vi "I2C Grove AlphaNumeric LED.vi"() -> ()   [LabVIEW 2020, in "CTI-Scratchpad.lvlib"]
uses:
  CTI-Scratchpad.lvlib
  CTI/Identity.ctl
  CTI/Error Reporting.ctl
  CTI/I2C Address.ctl
  CTI/GPIO Number.ctl
  CTI/I2C Number.ctl
  CTI/Session/Session.lvclass
  CTI-Peripheral/LEDAlphaNumeric/HT16K33 LED Driver/HT16K33 LED Driver.lvclass
  CTI/VisaComms/VisaComms.lvclass
  CTI/CTI.lvlib
panel:
  in  "Numeric In":string
  in  "Set Numeric":bool
  in  "String":string
  in  "Set Char":bool
  out "Identity":T1
  in  "stop":bool
  in  "Grove Connector":enum16{"I2C0", "I2C1"}(ring)
  out "error out":errorcluster
  in  "Port":refnum<visa-resource-name>="COM4"
  # "https://wiki.seeedstudio.com/Grove-0.54_inch_Red_Quad_Alphanumeric_Display/"
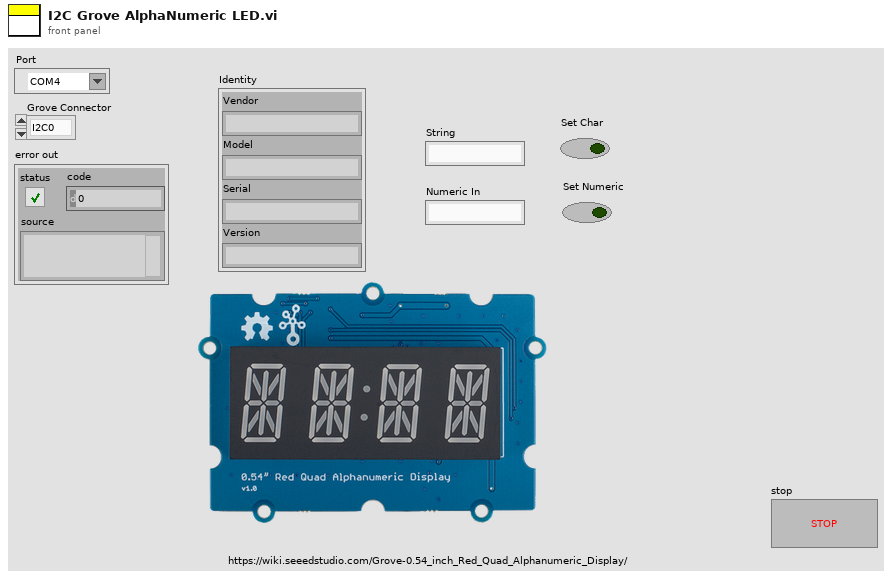
[diagram p1: front panel]
types:
  T1 = typedef "CTI.lvlib/Identity.ctl" = cluster{"Vendor":string, "Model":string, "Serial":string, "Version":string}
  T2 = typedef "CTI.lvlib/I2C Address.ctl" = u8
  T3 = typedef "CTI.lvlib/Error Reporting.ctl" = enum16{"Minimal", "Moderate", "Full"}
  T4 = typedef "CTI.lvlib/I2C Number.ctl" = i8
  T5 = typedef "CTI.lvlib/GPIO Number.ctl" = i8
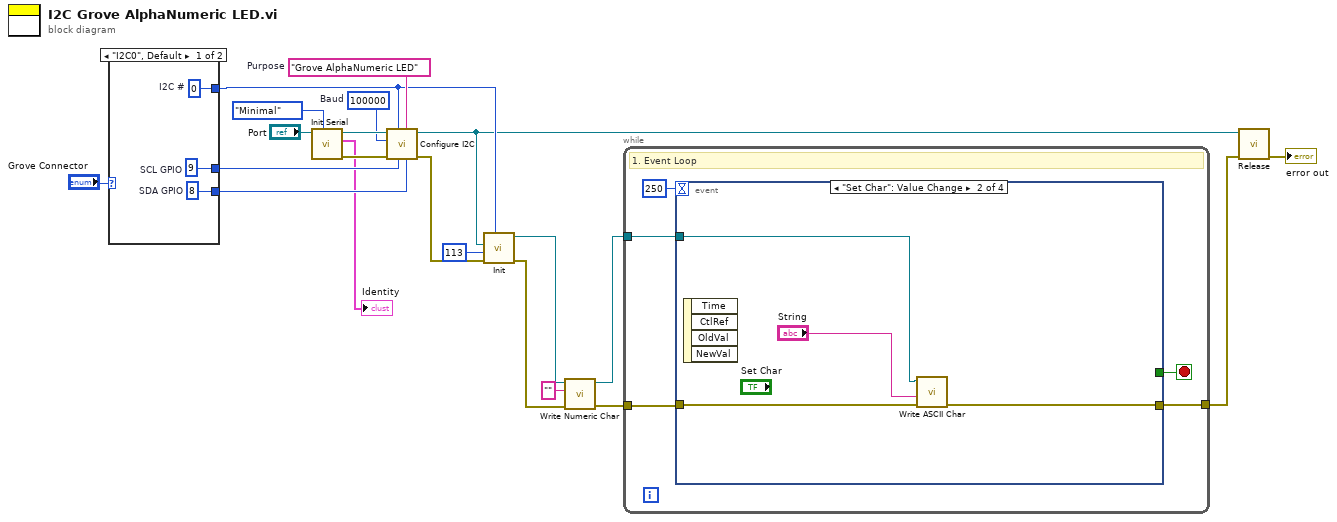
[diagram p0: block diagram]
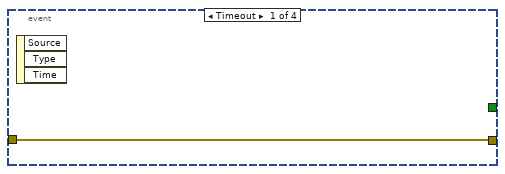
[diagram p2: hidden frame]
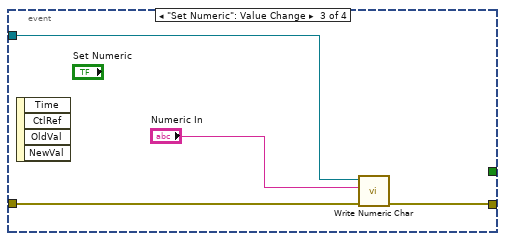
[diagram p3: hidden frame]
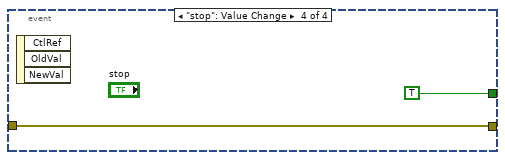
[diagram p4: hidden frame]
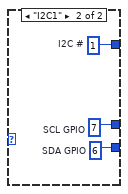
[diagram p5: hidden frame]
diagram:
  w16 = "Grove AlphaNumeric LED"  # Purpose
  w17 = u32 100000  # Baud
  n1 = case shown="\"I2C0\", Default" "Grove Connector" {
    tunnel: [w24 w27] -> w14
    tunnel: [w23 w26] -> w13
    tunnel: [w22 w25] -> w9
    frame "I2C0", Default {
      w22 = T4 0  # I2C #
      w23 = T5 8  # SDA GPIO
      w24 = T5 9  # SCL GPIO
    }
    frame "I2C1" {
      w25 = T4 1  # I2C #
      w26 = T5 6  # SDA GPIO
      w27 = T5 7  # SCL GPIO
    }
  }
  n2 = call "Init Serial.vi"("Error Checking (Full)"=Error_Reporting."Minimal", "VISA resource name in"="Port") -> ("error out"=w18:errorcluster, "Identity"=→"Identity":T1, "Session"=w19:refnum<class "Session.lvclass">)  [unwired: 7 in]
  n3 = call "Configure I2C.vi"("SDA GPIO"=w13, "Purpose (\"I2C\")"=w16, "SCL GPIO"=w14, "I2C #"=w9, "error in (no error)"=w18, "Baud"=w17, "Session in"=w19) -> ("error out"=w6:errorcluster, "Session out"=w8:refnum<class "Session.lvclass">)  [unwired: 3 in]
  n4 = call "Init.vi"("I2C #"=w9, "error in (no error)"=w6, "Address"=T2 113, "Session In"=w8) -> ("error out"=w4:errorcluster, "HT16K33 LED Driver Out"=w3:refnum<class "HT16K33 LED Driver.lvclass">)  [unwired: 6 in]
  n5 = call-dynamic "Write Numeric Char.vi"("error in (no error)"=w4, "Numeric In"="", "HT16K33 LED Driver  in"=w3) -> ("error out"=w5:errorcluster, "HT16K33 LED Driver out"=w1:refnum<class "HT16K33 LED Driver.lvclass">)  [unwired: 7 in]
  n6 = while {
    tunnel: w5 -> [w31]
    tunnel: [w30] -> w11
    tunnel: w1 -> [w32]
    stop <- w29 stop-if-true
    # "1. Event Loop"
    n7 = event shown="[1] \"Set Char\": Value Change" {
      selector: _ -> [_ _ _ _]
      dyn-events: _ -> [_ _ _ _]
      timeout: 250 -> [_ _ _ _]
      tunnel: w32 -> [_ w35 w41 _]
      tunnel: w31 -> [w33 w37 w40 w43]
      tunnel: [w33 w36 w39 w43] -> w30
      tunnel: [_ _ _ TRUE] -> w29
      event Timeout {
        n8 = event-data() -> ()  [unwired: 1 in, 3 out]
      }
      event "Set Char": Value Change {
        n9 = event-data() -> ()  [unwired: 1 in, 4 out]
        n10 = call-dynamic "Write ASCII Char.vi"("error in (no error)"=w37, "Char"="String", "HT16K33 LED Driver in"=w35) -> ("error out"=w36:errorcluster)  [unwired: 7 in, 1 out]
      }
      event "Set Numeric": Value Change {
        n11 = event-data() -> ()  [unwired: 1 in, 4 out]
        n12 = call-dynamic "Write Numeric Char.vi"("error in (no error)"=w40, "Numeric In"="Numeric In", "HT16K33 LED Driver  in"=w41) -> ("error out"=w39:errorcluster)  [unwired: 7 in, 1 out]
      }
      event "stop": Value Change {
        n13 = event-data() -> ()  [unwired: 1 in, 3 out]
      }
    }
  }
  n14 = call-dynamic "Release.vi"("error in (no error)"=w11, "Session in"=w8) -> ("error out"=→"error out":errorcluster)  [unwired: 9 in]
